vi "Barcode scanner lisen MIC.vi"(8 "error out 3":errorcluster, 10 "port":u16=1000, 11 "service name":string="192.168.1.20") -> (0 "error out 2":errorcluster, 2 "Exit":bool, 3 "data out":string)   [LabVIEW 2015]
uses:
  Galobal variable_TI.vi
panel:
  in  "stop":bool
  out "Numeric":i32
  out "error out":errorcluster
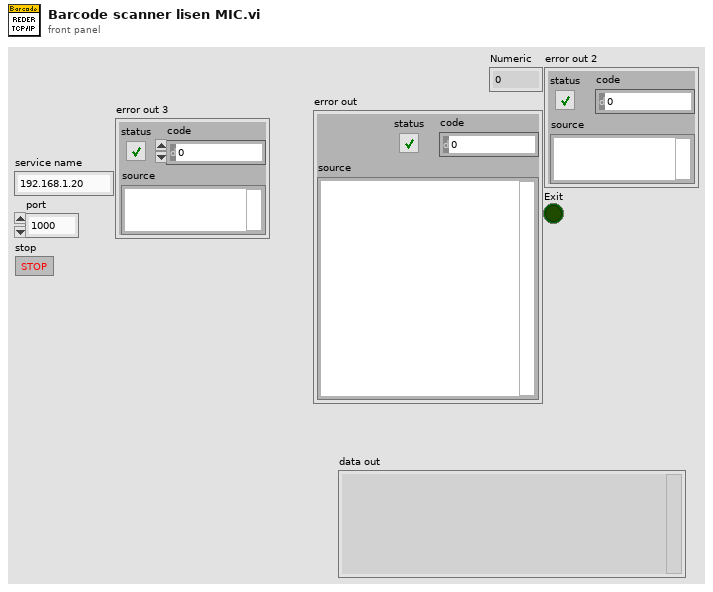
[diagram p1: front panel]
types:
  T1 = enum16{"Standard", "Buffered", "CRLF", "Immediate"}
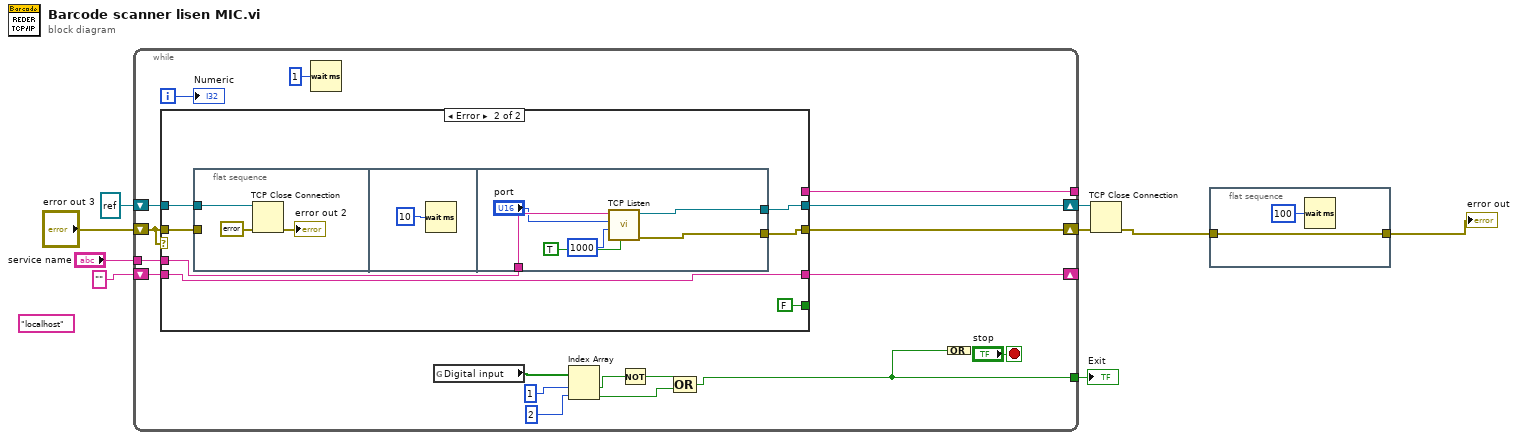
[diagram p0: block diagram]
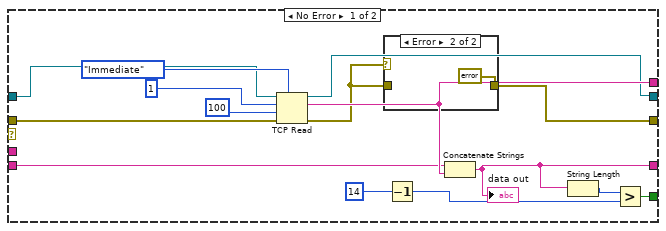
[diagram p2: hidden frame]
diagram:
  (unwired) "localhost" ("service name")
  n1 = while {
    tunnel: [w25] -> _
    shift-right: [w27] -> w9
    shift-left: refnum<k5> refnum ("connection ID") -> [w24]
    shift-right: [w26] -> w8
    shift-left: "error out 3" -> [w23]
    tunnel: "service name" -> [w22]
    shift-right: [w21] -> _
    shift-left: "" -> [w20]
    tunnel: [w11] -> w3
    i -> [w19]
    stop <- "stop" stop-if-true
    n2 = case shown="Error" w23 {
      tunnel: [w37 w47] -> w27
      tunnel: [w28 w46] -> w26
      tunnel: [w39 _] -> w25
      tunnel: w24 -> [w41 w51]
      tunnel: w23 -> [w40 w50]
      tunnel: w22 -> [_ w49]
      tunnel: [w35 w48] -> w21
      tunnel: w20 -> [w38 w48]
      tunnel: [w33 FALSE] -> _
      frame No Error {
        n3 = TCP Read(connection ID=w41, bytes to read=1, error in (no error)=w40, 7:T1."Immediate" ("mode (standard)"), 9:100 ("timeout ms (25000)")) -> (connection ID out=w37:refnum<k5>, data out=w39:string, error out=w29:errorcluster)
        n4 = case shown="Error" w29 {
          tunnel: [w43 errorcluster {"status"=FALSE, "code"=0, "source"=""} ("error out")] -> w28
          tunnel: w29 -> [w43 _]
          frame No Error {
          }
          frame Error {
          }
        }
        n5 = Decrement(x=14) -> (x-1=w31:i32)
        n6 = Concatenate Strings(w38, w39) -> (w35:string)
        "data out" <- w35
        n7 = String Length(string=w35) -> (length=w34:i32)
        n8 = Greater?(x=w34, y=w31) -> (0:w33:bool)
      }
      frame Error {
        n9 = flat-sequence {
          tunnel: w51 -> [w54]
          tunnel: w50 -> [_]
          tunnel: w49 -> [w60]
          tunnel: [w59] -> w47
          tunnel: [w58] -> w46
          frame #0 {
            n10 = TCP Close Connection(connection ID=w54, error in (no error)=errorcluster {"status"=FALSE, "code"=0, "source"=""}) -> (error out=→"error out 2":errorcluster)  [unwired: 1 in, 1 out]
          }
          frame #1 {
            n11 = Wait (ms)(milliseconds to wait=u32 10) -> ()  [unwired: 1 out]
          }
          frame #2 {
            n12 = call <vilib>:"TCP Listen.vi"("resolve remote address (T)"=TRUE, "timeout ms (wait forever: -1)"=1000, "port"="port", "service name"=w60) -> ("error out"=w58:errorcluster, "connection ID"=w59:refnum<k5>)  [unwired: 3 in, 3 out]
          }
        }
      }
    }
    n13 = Wait (ms)(milliseconds to wait=u32 1) -> ()  [unwired: 1 out]
    n14 = global read "Galobal variable_TI.vi" "Digital input"() -> (w17:bool[])
    n15 = Index Array(array=w17, index #1=1 ("index"), index #2=2 ("index")) -> (element #1=w14:bool, element #2=w12:bool)
    n16 = Not(x=w14) -> (.not. x?=w13:bool)
    n17 = Compound Arithmetic op=OR(w13, w12) -> (w11:bool)
    n18 = Compound Arithmetic op=OR(w11) -> ()  [unwired: 1 out]
    "Numeric" <- w19
  }
  "Exit" <- w3
  n19 = TCP Close Connection(connection ID=w9, error in (no error)=w8) -> (error out=w2:errorcluster)  [unwired: 1 in, 1 out]
  n20 = flat-sequence {
    tunnel: w2 -> [w63]
    tunnel: [w63] -> w1
    frame #0 {
      n21 = Wait (ms)(milliseconds to wait=u32 100) -> ()  [unwired: 1 out]
    }
  }
  "error out" <- w1
